vi "New.vi"(6 "Timeout ms (25000)":i32=25000, 8 "Error In":errorcluster, 9 "Local Port (61556)":u16=61556, 10 "Port (61557)":u16=61557, 11 "IP Address":string="127.0.0.1") -> (0 "Error Out":errorcluster, 3 "Sender Ref.":refnum<class "Sender.lvclass">)   [LabVIEW 2020, in "RemoteVariables.lvlib" / "Sender.lvclass"]
uses:
  Sender.lvclass
  Sender.lvclass/Sender.ctl
  UDP/UDP.lvclass
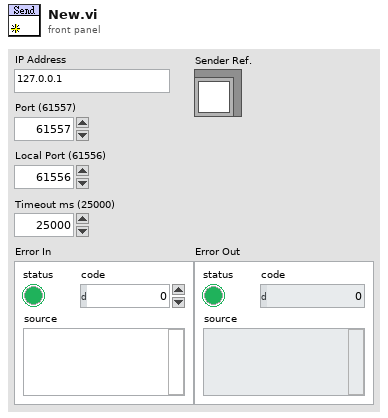
[diagram p1: front panel]
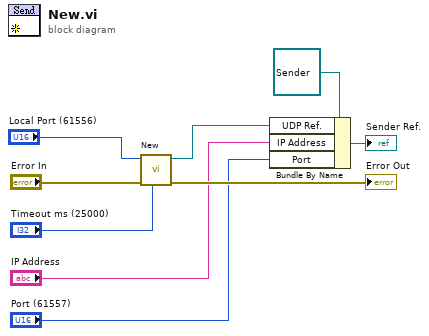
[diagram p0: block diagram]
diagram:
  n1 = call "New.vi"("Timeout ms (25000)"="Timeout ms (25000)", "Error In"="Error In", "Port (61557)"="Local Port (61556)") -> ("Error Out"=→"Error Out":errorcluster, "UDP Ref."=w7:refnum<class "UDP.lvclass">)  [unwired: 7 in]
  n2 = Bundle By Name(cluster=refnum<class "Sender.lvclass"> refnum ("RemoteVariables.lvlib:Sender.lvclass"), "UDP Ref."=w7, "IP Address"="IP Address", "Port"="Port (61557)") -> (→"Sender Ref.":refnum<class "Sender.lvclass">)
